vi "readBuffer.vi"(8 "error in (no error)":errorcluster, 10 "byte count":u32, 11 "UART Actor in":refnum<class "UART Actor.lvclass">) -> (0 "error out":errorcluster, 3 "UART Actor out":refnum<class "UART Actor.lvclass">)   [LabVIEW 2020, in "UART Actor.lvlib" / "UART Actor.lvclass"]
uses:
  UART Actor.lvclass
  UART Actor.lvclass/UART Actor.ctl
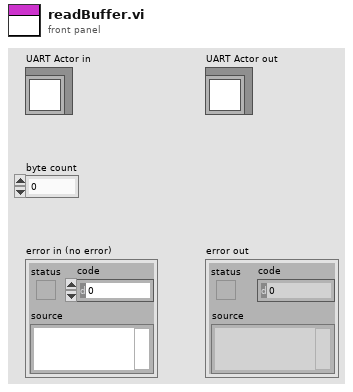
[diagram p1: front panel]
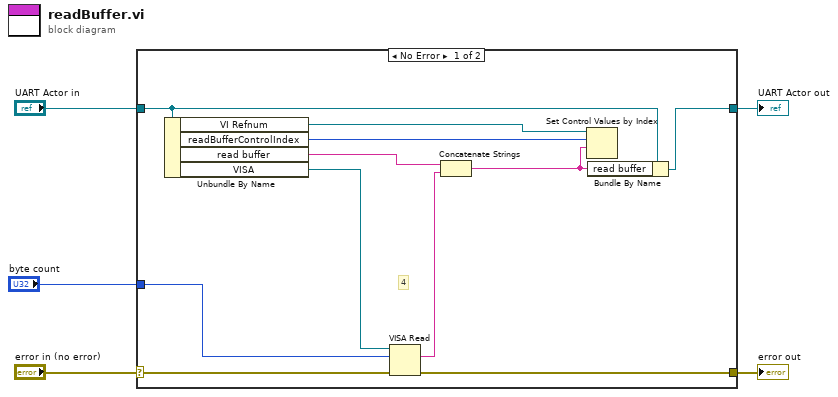
[diagram p0: block diagram]
diagram:
  n1 = case shown="No Error" "error in (no error)" {
    selector: "error in (no error)" -> [w15 w18]
    tunnel: [w14 w18] -> w4
    tunnel: [w10 w17] -> w2
    tunnel: "UART Actor in" -> [w9 w17]
    tunnel: "byte count" -> [w12 _]
    frame No Error {
      # "4"
      n2 = Unbundle By Name(w9) -> ("VI Refnum"=w7:refnum<vi>, "readBufferControlIndex"=w8:i32, "read buffer"=w11:string, "VISA"=w13:refnum<visa-resource-name>)
      n3 = VISA Read(VISA resource name=w13, byte count=w12, error in (no error)=w15) -> (read buffer=w16:string, error out=w14:errorcluster)  [unwired: 2 out]
      n4 = Concatenate Strings(w11, w16) -> (w6:string)
      n5 = Set Control Values by Index(0:w7, 1:w8, 2:w6) -> ()  [unwired: 1 in, 1 out]
      n6 = Bundle By Name(cluster=w9, "read buffer"=w6) -> (w10:refnum<class "UART Actor.lvclass">)
    }
    frame Error {
    }
  }
  "error out" <- w4
  "UART Actor out" <- w2
